vi "SteerOptimizer.vi"(7 "Current Heading":dbl(slide) scale=-20.0..20.0, 9 "Throttle":dbl, 10 "Setpoint":dbl(knob) scale=-3.1415..3.1415) -> (0 "Inverted":bool, 1 "Throttle out":dbl, 2 "Heading":dbl(slide) scale=-20.0..20.0)   [LabVIEW 2018]
uses:
  <vilib>/Analysis/coordinate.llb/Angle Range (Degree).ctl
  <vilib>/Analysis/coordinate.llb/Wrap Angle (scalar).vi
  <vilib>/Analysis/NI_AAL_Angle.lvlib
panel:
  out "Heading":dbl(knob) scale=-3.1415..3.1415
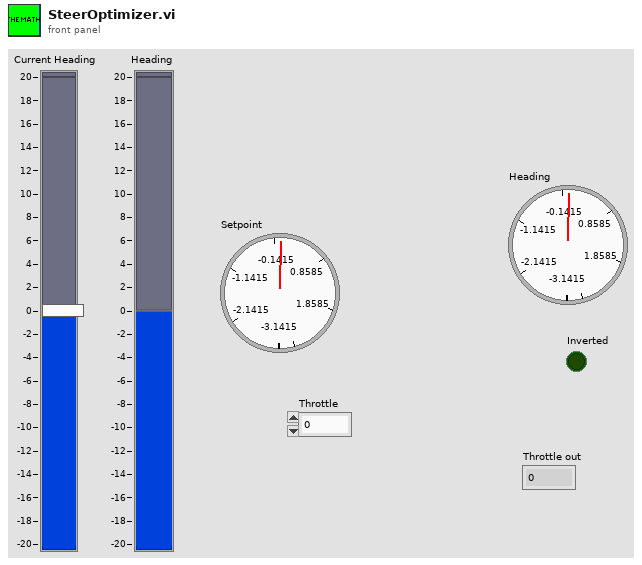
[diagram p1: front panel]
types:
  T1 = typedef "NI_AAL_Angle.lvlib/Angle Range (Degree).ctl" = u16
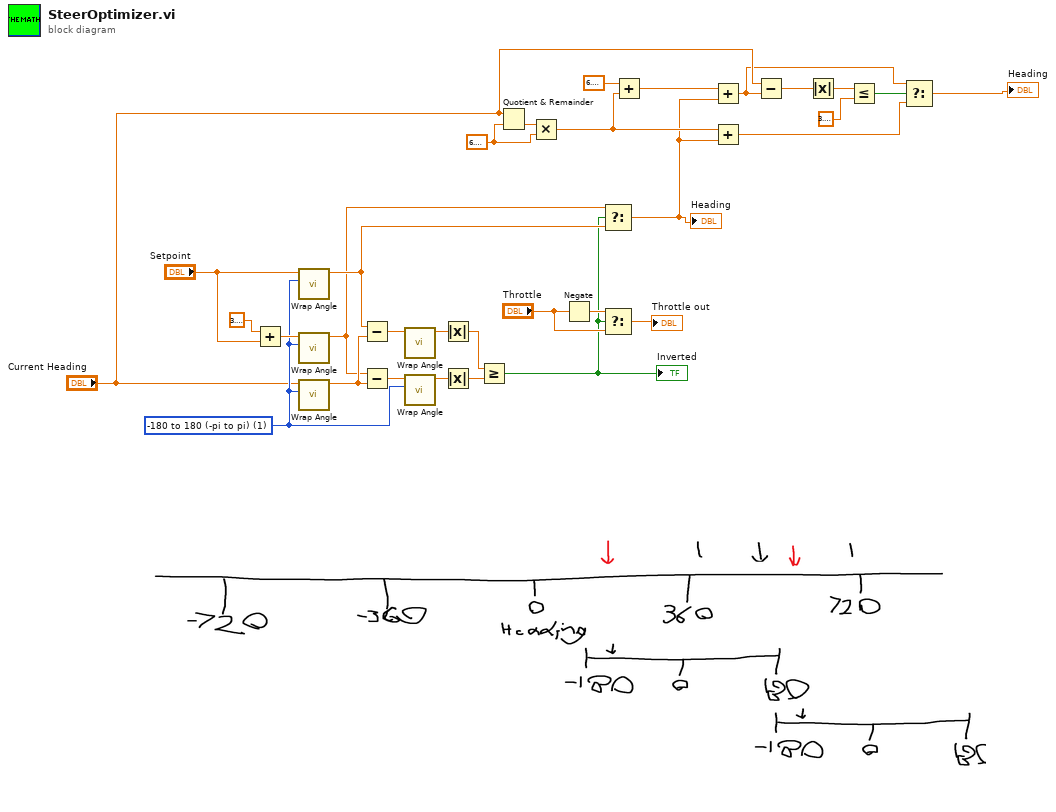
[diagram p0: block diagram]
diagram:
  w19 = 6.283185307179586
  w10 = T1 1 items=["none", "-180 to 180 (-pi to pi)", "0 to 360 (0 to 2pi)"] ("angle range")
  n1 = Add(x=3.141592653589793, y="Setpoint") -> (x+y=w25:dbl)
  n2 = call-poly <vilib>:"Wrap Angle.vi"("angle range"=w10, "angle in"="Setpoint") -> ("angle out"=w16:dbl)  [unwired: 8 in, 1 out]
  n3 = call-poly <vilib>:"Wrap Angle.vi"("angle range"=w10, "angle in"=w25) -> ("angle out"=w15:dbl)  [unwired: 8 in, 1 out]
  n4 = call-poly <vilib>:"Wrap Angle.vi"("angle range"=w10, "angle in"="Current Heading") -> ("angle out"=w23:dbl)  [unwired: 8 in, 1 out]
  n5 = Subtract(x=w16, y=w23) -> (x-y=w18:dbl)
  n6 = Subtract(x=w15, y=w23) -> (x-y=w17:dbl)
  n7 = call-poly <vilib>:"Wrap Angle.vi"("angle in"=w18) -> ("angle out"=w28:dbl)  [unwired: 9 in, 1 out]
  n8 = call-poly <vilib>:"Wrap Angle.vi"("angle range"=w10, "angle in"=w17) -> ("angle out"=w27:dbl)  [unwired: 8 in, 1 out]
  n9 = Absolute Value(x=w28) -> (abs(x)=w30:dbl)
  n10 = Absolute Value(x=w27) -> (abs(x)=w31:dbl)
  n11 = Greater Or Equal?(x=w30, y=w31) -> (x >= y?=w1:bool)
  "Inverted" <- w1
  n12 = Quotient & Remainder(x="Current Heading", y=w19) -> (floor(x/y)=w20:dbl)  [unwired: 1 out]
  n13 = Multiply(x=w20, y=w19) -> (x*y=w12:dbl)
  n14 = Negate(x="Throttle") -> (-x=w22:dbl)
  n15 = Select(t=w15, s=w1, f=w16) -> (s? t:f=w11:dbl)
  "Heading" <- w11
  n16 = Select(t=w22, s=w1, f="Throttle") -> (s? t:f=→"Throttle out":dbl)
  n17 = Add(x=6.283185307179586, y=w12) -> (x+y=w13:dbl)
  n18 = Add(x=w13, y=w11) -> (x+y=w2:dbl)
  n19 = Add(x=w12, y=w11) -> (x+y=w3:dbl)
  n20 = Subtract(x="Current Heading", y=w2) -> (x-y=w6:dbl)
  n21 = Absolute Value(x=w6) -> (abs(x)=w9:dbl)
  n22 = Less Or Equal?(x=w9, y=3.141592653589793) -> (x <= y?=w7:bool)
  n23 = Select(t=w2, s=w7, f=w3) -> (s? t:f=→"Heading":dbl)
